vi "ASK_GenVioce.vi"(7 "write_filename":string, 8 "error in (no error)":errorcluster caption="错误输入（无错误）", 9 "sampleVal":dbl format="%#_13g", 10 "还原后数据":dbl[](array[numeric]) format="%#_13g", 11 "PathIn":path) -> (0 "error out":errorcluster caption="错误输出", 1 "数组":dbl[](array[numeric]) format="%#_13g", 3 "PathOut":path)   [LabVIEW 2015]
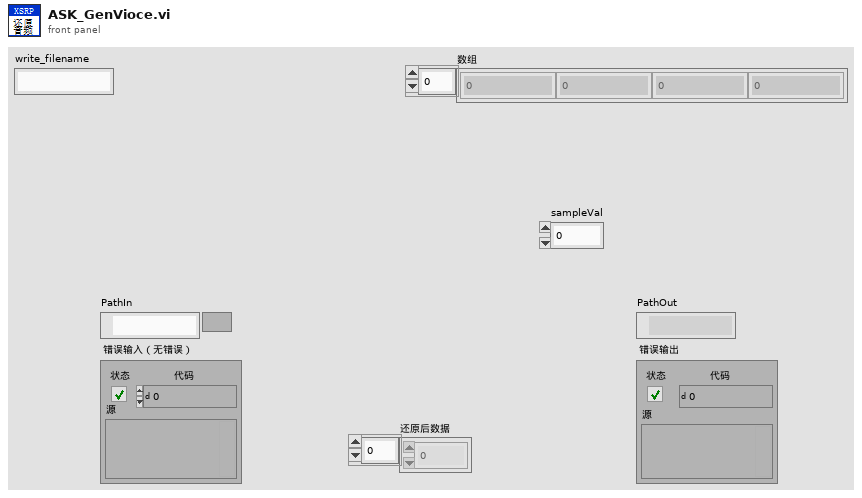
[diagram p1: front panel]
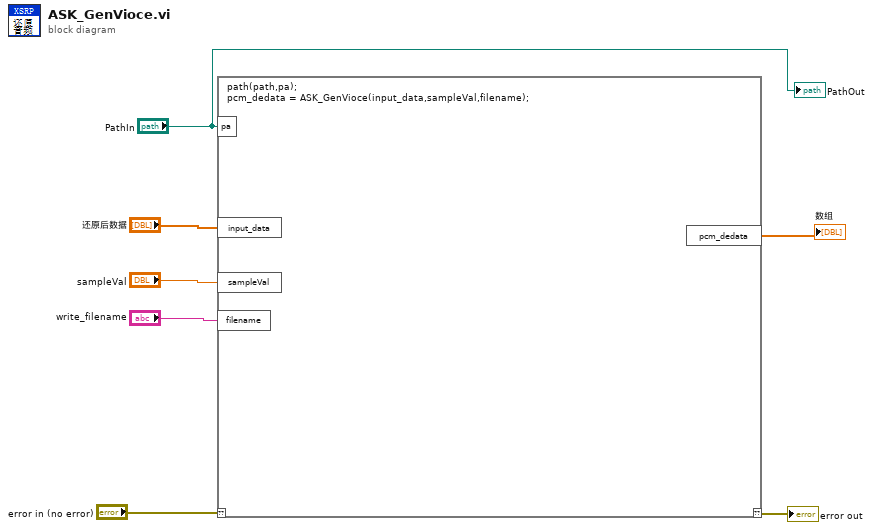
[diagram p0: block diagram]
diagram:
  n1 = script code="path(path,pa);\npcm_dedata = ASK_GenVioce(input_data,sampleVal,filename);"("??"="error in (no error)", "pa"="PathIn", "input_data"="还原后数据", "sampleVal"="sampleVal", "filename"="write_filename") -> ("??"=→"error out":errorcluster, "pcm_dedata"=→"数组":dbl[])
  "PathOut" <- "PathIn"
